vi "AcquireVandA.vi"(7 "error in (no error)":errorcluster caption="错误输入（无错误）", 10 "Hardware Configuration":T1 caption="硬件配置") -> (0 "error out":errorcluster caption="错误输出", 2 "Graph Data":waveform(dbl)[](array[waveform]) caption="图形数据")   [LabVIEW 2014, in "Acquisitions.lvlib"]
doc: "按硬件配置输入中的信号类型，生成采样波形。"
uses:
  Acquisitions.lvlib
  HW Configuration.ctl
  <vilib>/DAQmx/read.llb/DAQmx Read (Analog 1D Wfm NChan NSamp).vi
  <vilib>/DAQmx/create/channels.llb/DAQmx Create Channel (AI-Voltage-Basic).vi
  <vilib>/DAQmx/configure/timing.llb/DAQmx Timing (Sample Clock).vi
  <vilib>/DAQmx/miscellaneous.llb/DAQmx Fill In Error Info.vi
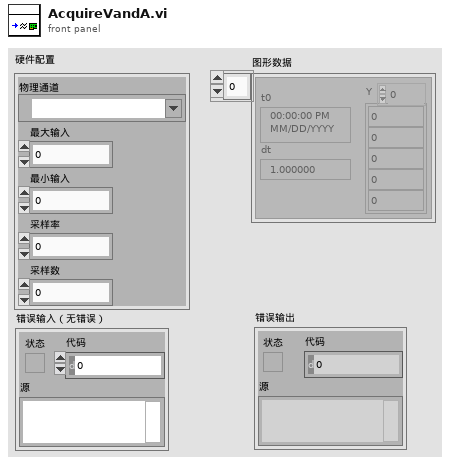
[diagram p1: front panel]
types:
  T1 = typedef "Acquisitions.lvlib/HW Configuration.ctl" = cluster{"Physical Channel":tag, "Maximum Input":dbl, "Minimum Input":dbl, "Sample Rate":dbl, "Number of Samples":i32}
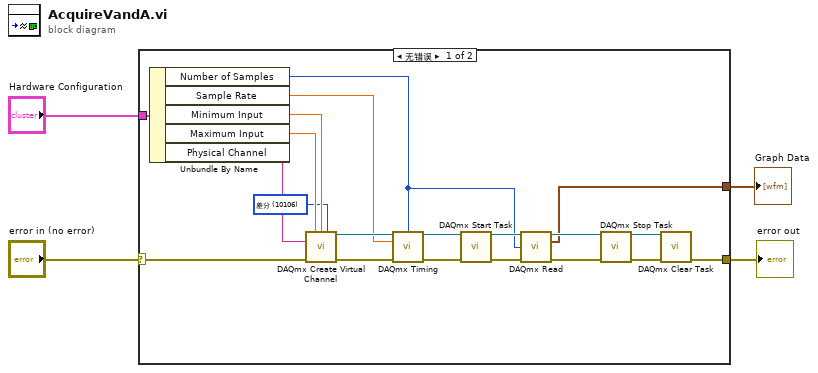
[diagram p0: block diagram]
diagram:
  n1 = case shown="无错误" "error in (no error)" {
    selector: "error in (no error)" -> [w15 w25]
    tunnel: [w16 w25] -> w3
    tunnel: "Hardware Configuration" -> [w24 _]
    tunnel: [w19 _] -> w1
    frame No Error {
      w5 = 10106 items=["默认"=-1, "RSE"=10083, "NRSE"=10078, "差分"=10106, "伪差分"=12529] ("input terminal configuration")
      n2 = Unbundle By Name(w24) -> ("Number of Samples"=w6:i32, "Sample Rate"=w9:dbl, "Minimum Input"=w12:dbl, "Maximum Input"=w13:dbl, "Physical Channel"=w14:tag)
      n3 = call-poly <vilib>:"DAQmx Create Virtual Channel.vi"("maximum value"=w13, "minimum value"=w12, "input terminal configuration"=w5, "physical channels"=w14, "error in"=w15) -> ("task out"=w10:refnum<k21>, "error out"=w11:errorcluster)  [unwired: 9 in]
      n4 = call-poly <vilib>:"DAQmx Timing.vi"("task/channels in"=w10, "samples per channel"=w6, "rate"=w9, "error in"=w11) -> ("task out"=w8:refnum<k21>, "error out"=w7:errorcluster)  [unwired: 10 in]
      n5 = call <vilib>:"DAQmx Start Task.vi"("task/channels in"=w8, "error in"=w7) -> ("task out"=w23:refnum<k21>, "error out"=w22:errorcluster)  [unwired: 12 in]
      n6 = call-poly <vilib>:"DAQmx Read.vi"("task/channels in"=w23, "number of samples per channel"=w6, "error in"=w22) -> ("task out"=w20:refnum<k21>, "data"=w19:waveform(dbl)[], "error out"=w21:errorcluster)  [unwired: 10 in]
      n7 = call <vilib>:"DAQmx Stop Task.vi"("task/channels in"=w20, "error in"=w21) -> ("task out"=w17:refnum<k21>, "error out"=w18:errorcluster)  [unwired: 12 in]
      n8 = call <vilib>:"DAQmx Clear Task.vi"("task in"=w17, "error in"=w18) -> ("error out"=w16:errorcluster)  [unwired: 13 in]
    }
    frame Error {
    }
  }
  "error out" <- w3
  "Graph Data" <- w1
